vi "Sub Panel Control.vi"(8 "에러 입력":errorcluster caption="에러 입력(에러 없음)", 11 "서브패널 배열":refnum<vi>[](array[refnum])) -> (0 "에러 출력":errorcluster, 3 "VI참조":refnum<vi>[](array[refnum]))   [LabVIEW 2020]
uses:
  Controls/Cmd_File path.ctl
  Controls/Cmd_File Type.ctl
  <vilib>/Utility/error.llb/DialogType.ctl
  Variables/Global_Cal Info.vi
  <vilib>/Utility/error.llb/Error Cluster From Error Code.vi
  <vilib>/ErrorRing/Error Ring.xnode
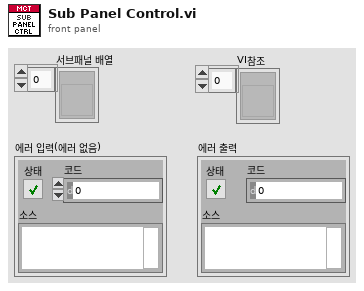
[diagram p1: front panel]
types:
  T1 = typedef "Cmd_File Type.ctl" = enum16{"엑셀", "엑셀(2003)", "텍스트", "설정", "2진", "VI", "CSV", "LOG", "폴더"}
  T2 = typedef "Cmd_File path.ctl" = enum16{"에러로그", "데이터파일경로", "성적서원본", "지난성적서", "Data Files", "경로생성", "Updater", "Template", "설정파일경로", "FTP Upload", "Update 경로", "어플리케이션"}
  T3 = enum32{"Bad", "Idle", "Run top level", "Running"}
  T4 = typedef "DialogType.ctl" = u16
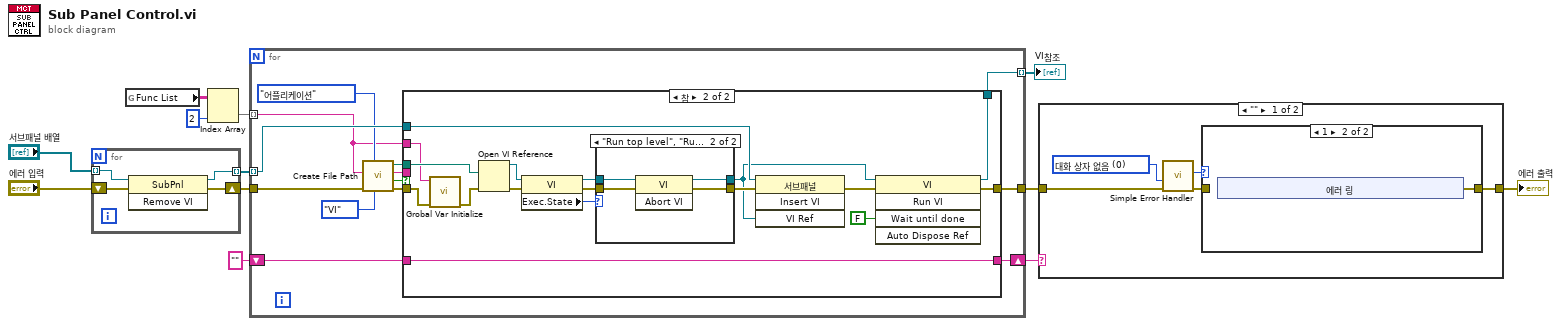
[diagram p0: block diagram]
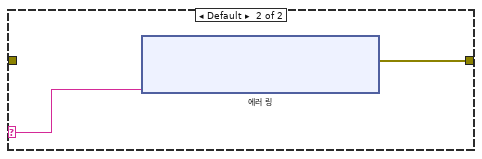
[diagram p3: hidden frame]
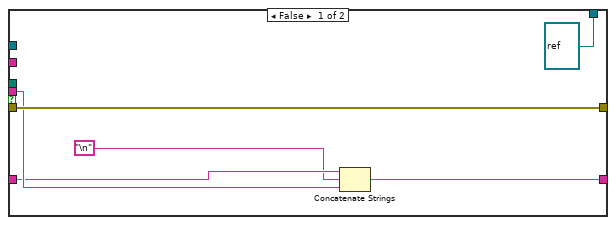
[diagram p4: hidden frame]
diagram:
  n1 = for {
    tunnel: "서브패널 배열" -> [w15] mode=indexing
    shift-right: [w14] -> w9
    shift-left: "에러 입력" -> [w16]
    tunnel: [w13] -> w10 mode=indexing
    n2 = invoke class="SubPnl" method="Remove VI"(reference=w15, error in=w16) -> (reference out=w13:refnum<vi>, error out=w14:errorcluster)  [unwired: 1 in, 1 out]
  }
  n3 = global read "Global_Cal Info.vi" "Func List"() -> (w4:string[][])
  n4 = Index Array(array=w4, index (col)=2 ("비활성화된 인덱스 (열)")) -> (element=w11:string[])  [unwired: 1 in]
  n5 = for {
    tunnel: w10 -> [w29] mode=indexing
    tunnel: w11 -> [w18] mode=indexing
    tunnel: w9 -> [w25]
    tunnel: [w28] -> w3
    shift-right: [w26] -> w6
    shift-left: "" -> [w27]
    tunnel: [w17] -> w1 mode=indexing
    n6 = call "Create File Path.vi"("파일타입"=Cmd_File_Type."VI", "항목"=Cmd_File_path."어플리케이션", "에러 입력"=w25, "문자열 in"=w18) -> ("error out"=w20:errorcluster, "파일존재?"=w21:bool, "문자열 out"=w22:string, "파일경로"=w23:path)  [unwired: 4 in]
    n7 = case shown="참" w21 {
      tunnel: w29 -> [_ w50]
      tunnel: [w35 w49] -> w28
      tunnel: w20 -> [w35 w39]
      tunnel: w23 -> [_ w48]
      tunnel: w22 -> [w34 _]
      tunnel: w27 -> [w33 w40]
      tunnel: [w32 w40] -> w26
      tunnel: w18 -> [_ w37]
      tunnel: [refnum<vi> refnum ("vi reference") w36] -> w17
      frame False {
        n8 = Concatenate Strings(w33, "\n", w34) -> (w32:string)
      }
      frame True {
        n9 = call "Grobal Var Initialize.vi"("에러 입력"=w39, "Func_ext"=w37) -> ("에러 출력"=w38:errorcluster)  [unwired: 9 in]
        n10 = Open VI Reference(vi path=w48, error in (no error)=w38) -> (vi reference=w46:refnum<vi>, error out=w47:errorcluster)  [unwired: 4 in]
        n11 = property class="VI"(reference=w46, error in=w47) -> (reference out=w44:refnum<vi>, error out=w45:errorcluster, "Exec.State"=w42:T3)
        n12 = case shown="\"Run top level\", \"Running\"" w42 {
          tunnel: w45 -> [w54 w58]
          tunnel: [w54 w56] -> w43
          tunnel: w44 -> [w53 w57]
          tunnel: [w53 w55] -> w41
          frame Default {
          }
          frame "Run top level", "Running" {
            n13 = invoke on="인보크 노드" class="VI" method="Abort VI"(reference=w57, error in=w58) -> (reference out=w55:refnum<vi>, error out=w56:errorcluster)  [unwired: 1 in, 1 out]
          }
        }
        n14 = invoke on="인보크 노드" class="서브패널" method="Insert VI"(reference=w50, error in=w43, "VI Ref"=w41) -> (error out=w51:errorcluster)  [unwired: 1 in, 3 out]
        n15 = invoke on="인보크 노드" class="VI" method="Run VI"(reference=w41, error in=w51, "Wait until done"=FALSE ("완료될 때까지 기다림")) -> (reference out=w36:refnum<vi>, error out=w49:errorcluster)  [unwired: 2 in, 3 out]
      }
    }
  }
  "VI참조" <- w1
  n16 = case shown="\"\"" w6 {
    selector: w6 -> [_ w71]
    tunnel: w3 -> [w63 _]
    tunnel: [w61 w72] -> w2
    frame "" {
      w59 = T4 0 items=["대화 상자 없음", "확인 메시지", "메시지 지속 또는 정지", "확인 메시지 + 경고", "지속/정지 + 경고"] ("type of dialog (OK msg:1)")
      n17 = call <vilib>:"Simple Error Handler.vi"("type of dialog (OK msg:1)"=w59, "error in (no error)"=w63) -> ("code out"=w62:i32, "error out"=w60:errorcluster)  [unwired: 3 in, 3 out]
      n18 = case shown="1" w62 {
        tunnel: [w64 w65] -> w61
        tunnel: w60 -> [w64 _]
        frame Default {
        }
        frame 1 {
          n19 = xnode "에러 링"() -> ("에러 출력"=w65:errorcluster)
        }
      }
    }
    frame Default {
      n20 = xnode "에러 링"("파라미터 0"=w71) -> ("에러 출력"=w72:errorcluster)
    }
  }
  "에러 출력" <- w2
